vi "SR_FFT_Biegebalken_a_v_s.vi"() -> ()   [LabVIEW 2012]
uses:
  <vilib>/express/express shared/transition.llb/Dynamic To Waveform Array.vi
  <vilib>/express/express shared/transition.llb/Waveform Array To Dynamic.vi
  <vilib>/express/express arith-compare/Formula/Block/exnFormulaBlock how many pts in the wave.vi
  <vilib>/express/express shared/ex_Modify Signal Name.vi
  <vilib>/express/express analysis/Spectral/Block/exnSpectralBlock spectral measurements peak poly.vi
  <vilib>/express/express analysis/Spectral/Block/exnSpectralBlock spectral measurements peak DDT.vi
  <vilib>/express/express arith-compare/Formula/XNode/ExpressFormulaBlockNode.xnode
  <vilib>/express/express analysis/Spectral/XNode/ExpressSpectralMeasurementsBlockNode.xnode
panel:
  out "Signalverlaufsgraph 3":dynamicdata(graph)
  out "Signalverlaufsgraph 2":dynamicdata(graph)
  out "Signalverlaufsgraph":dynamicdata(graph)
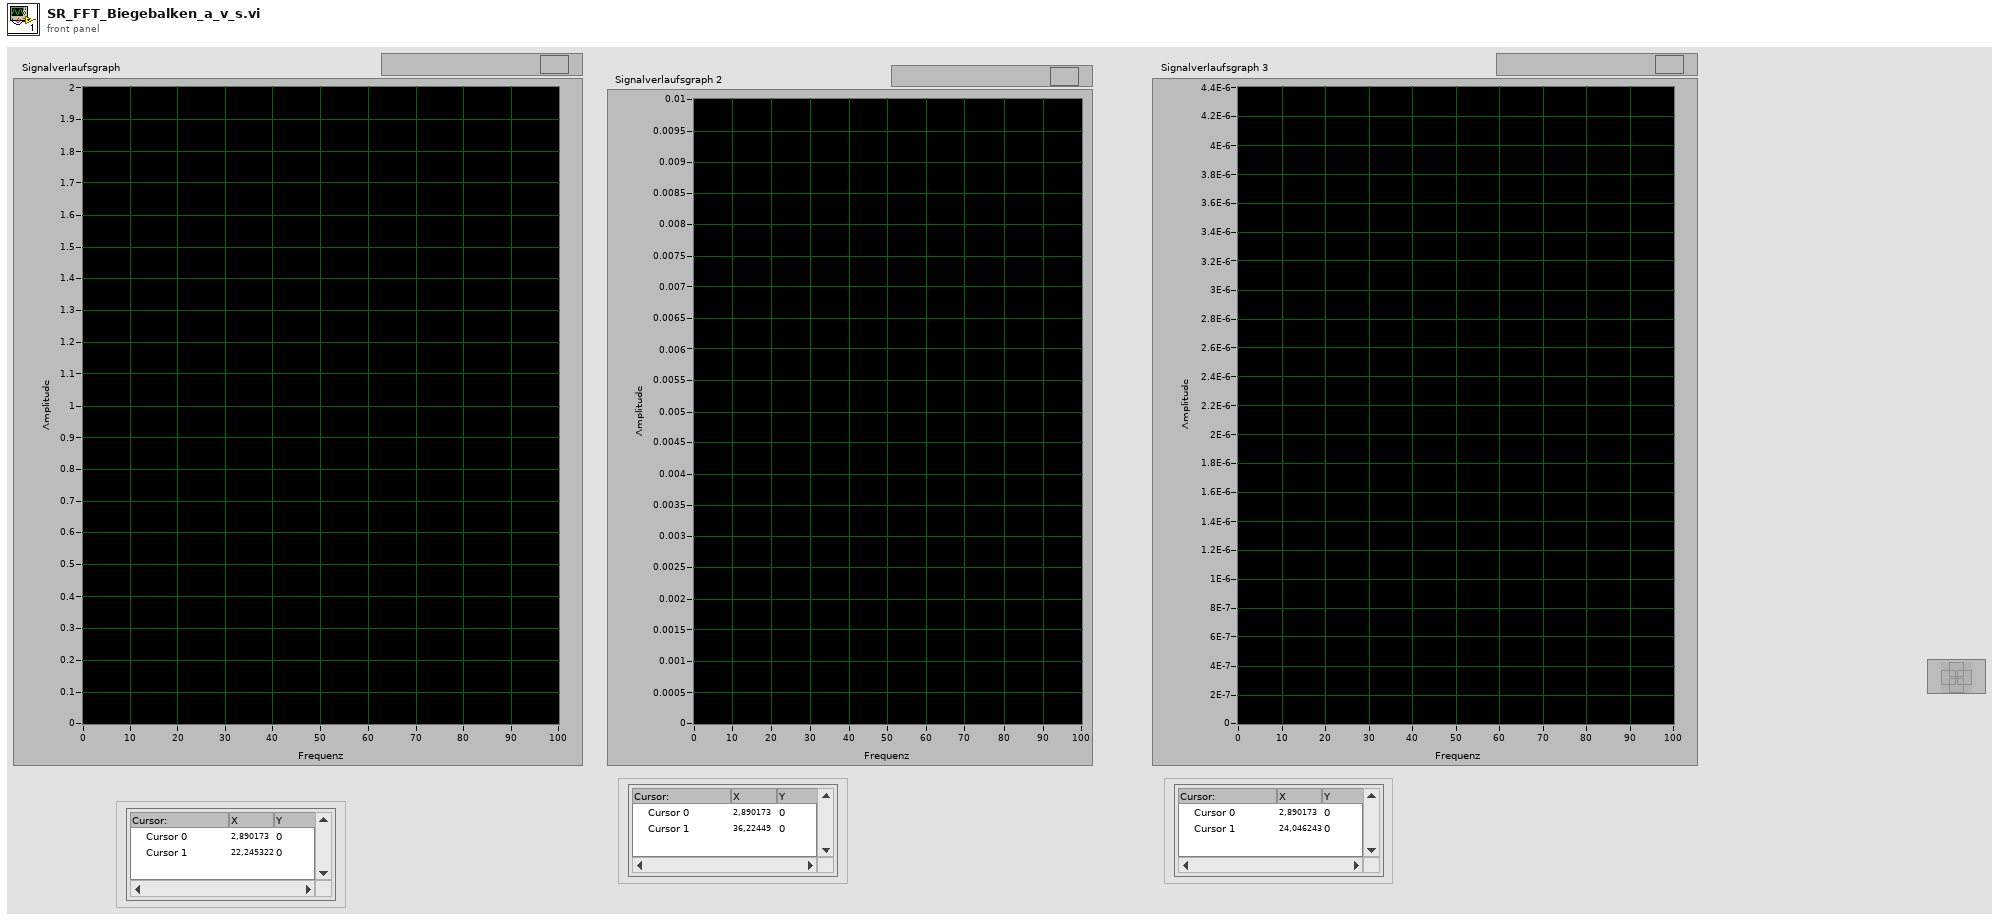
[diagram p1: front panel]
types:
  T1 = cluster{"averaging mode":u16, "weighting mode":u16, "number of averages":u32}
  T2 = cluster{"dB On (F)":bool, "unwrap phase (F)":bool, "convert to degree (F)":bool}
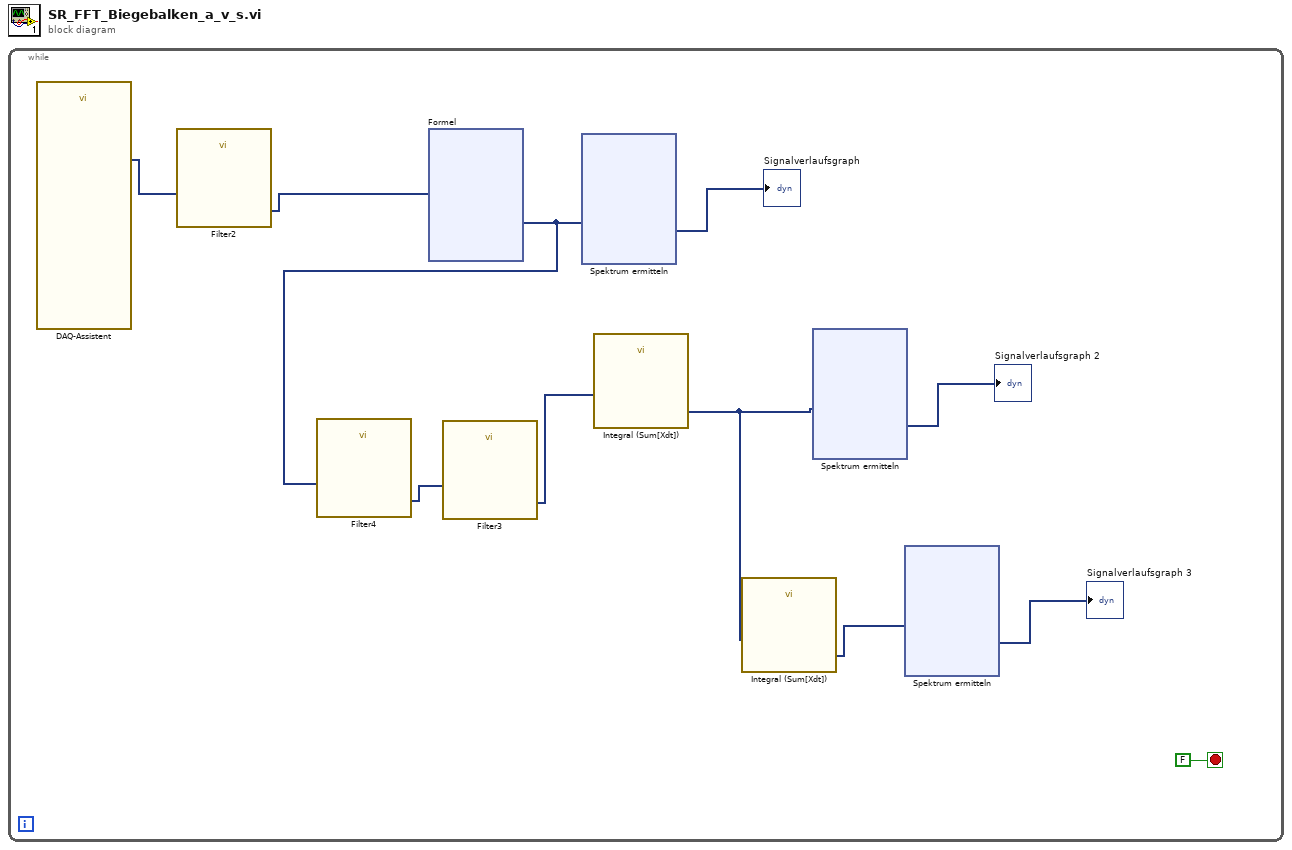
[diagram p0: block diagram]
diagram:
  n1 = while {
    stop <- FALSE stop-if-true
    n2 = call "DAQ-Assistent"() -> ("data"=w9:dynamicdata)  [unwired: 16 in, 3 out]
    n3 = call "Filter2"("Signal"=w9) -> ("Filtered Signal"=w1:dynamicdata)  [unwired: 9 in, 1 out]
    n4 = xnode "Formel"("X1"=w1) -> ("Ergebnis"=w3:dynamicdata)  [unwired: 1 in, 1 out]
    n5 = call "Filter4"("Signal"=w3) -> ("Filtered Signal"=w4:dynamicdata)  [unwired: 9 in, 1 out]
    n6 = call "Filter3"("Signal"=w4) -> ("Filtered Signal"=w2:dynamicdata)  [unwired: 9 in, 1 out]
    n7 = xnode "Spektrum ermitteln"("Signale"=w3) -> ("FFT - (Spitze)"=→"Signalverlaufsgraph":dynamicdata)  [unwired: 1 in, 2 out]
    n8 = call "Integral (Sum[Xdt])"("Signals"=w2) -> ("Result"=w6:dynamicdata)  [unwired: 5 in, 1 out]
    n9 = call "Integral (Sum[Xdt])"("Signals"=w6) -> ("Result"=w5:dynamicdata)  [unwired: 5 in, 1 out]
    n10 = xnode "Spektrum ermitteln"("Signale"=w6) -> ("FFT - (Spitze)"=→"Signalverlaufsgraph 2":dynamicdata)  [unwired: 1 in, 2 out]
    n11 = xnode "Spektrum ermitteln"("Signale"=w5) -> ("FFT - (Spitze)"=→"Signalverlaufsgraph 3":dynamicdata)  [unwired: 1 in, 2 out]
  }
